vi "uA_daq_gain_caculator.vi"(0 "Waveform Chart in":waveform(sgl), 5 "Calib_value":dbl, 9 "Range - Shunts":T1) -> (4 "Waveform out":waveform(dbl))   [LabVIEW 2015]
uses:
  Range_Shunt_selector.ctl
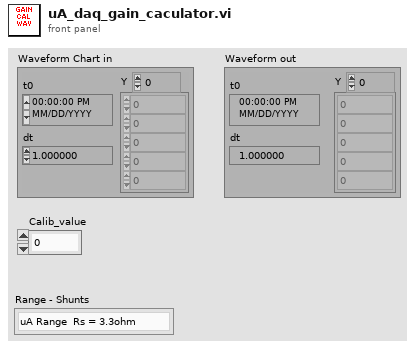
[diagram p1: front panel]
types:
  T1 = typedef "Range_Shunt_selector.ctl" = enum16{"uA Range  Rs = 3.3ohm", "mA Range Rs = 3.3Ohm", "mA Range Rs = 1Ohm", "mA Range Rs = 1Ohm - X2"}
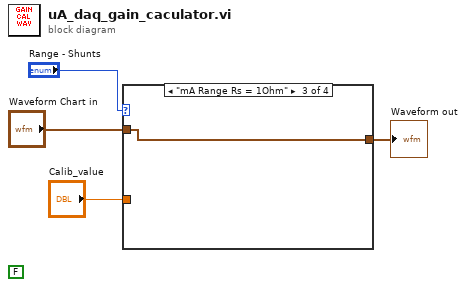
[diagram p0: block diagram]
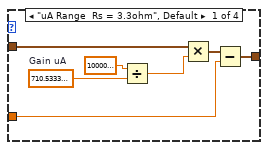
[diagram p2: hidden frame]
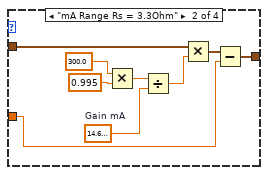
[diagram p3: hidden frame]
diagram:
  (unwired) FALSE ("s")
  n1 = case shown="\"mA Range Rs = 1Ohm\"" "Range - Shunts" {
    tunnel: "Waveform Chart in" -> [w9 w15 w21 w22]
    tunnel: [w5 w13 w21 w22] -> w1
    tunnel: "Calib_value" -> [w6 w12 _ _]
    frame "uA Range  Rs = 3.3ohm", Default {
      w10 = sgl 710.5333  # Gain uA
      n2 = Divide(x=sgl 1000000.0, y=w10) -> (x/y=w8:sgl)
      n3 = Multiply(x=w9, y=w8) -> (x*y=w7:waveform(sgl))
      n4 = Subtract(x=w7, y=w6) -> (x-y=w5:waveform(dbl))
    }
    frame "mA Range Rs = 3.3Ohm" {
      w19 = sgl 14.6  # Gain mA
      n5 = Multiply(x=300.0, y=0.995 ("Numeric")) -> (x*y=w20:dbl)
      n6 = Divide(x=w20, y=w19) -> (x/y=w16:dbl)
      n7 = Multiply(x=w15, y=w16) -> (x*y=w14:waveform(dbl))
      n8 = Subtract(x=w14, y=w12) -> (x-y=w13:waveform(dbl))
    }
    frame "mA Range Rs = 1Ohm" {
    }
    frame "mA Range Rs = 1Ohm - X2" {
    }
  }
  "Waveform out" <- w1
